vi "SWERVE_DRIVE_ACT.vi"(8 "in Swerve Module States":T4[](array[typedef]) {"Angle"."SIN" format="%13.4f"; "Angle"."COS" format="%13.4f"; "Angle"."VALUE" format="%13.4f"}, 9 "Gyro_Continuous_Rad":dbl, 10 "Swerve Drive Device Reference":T6[](array[typedef]), 11 "in SWERVE_DRIVE_KINEMATICS":T1 {"SavedModuleStates"."Angle"."SIN" format="%13.4f"; "SavedModuleStates"."Angle"."COS" format="%13.4f"; "SavedModuleStates"."Angle"."VALUE" format="%13.4f"; "PrevCoR"."Y" format="%14.3f"; "PrevCoR"."X" format="%14.3f"; "Modules"."Y" format="%14.3f"; "Modules"."X" format="%14.3f"}) -> (3 "out SWERVE_DRIVE_KINEMATICS":T1 {"SavedModuleStates"."Angle"."SIN" format="%13.4f"; "SavedModuleStates"."Angle"."COS" format="%13.4f"; "SavedModuleStates"."Angle"."VALUE" format="%13.4f"; "PrevCoR"."Y" format="%14.3f"; "PrevCoR"."X" format="%14.3f"; "Modules"."Y" format="%14.3f"; "Modules"."X" format="%14.3f"})   [LabVIEW 2019]
uses:
  <vilib>/Rock Robotics/WPI/ThirdParty/JAS_Junk/TrajLib/TypeDef/SWERVE_DRIVE_KINEMATICS.ctl
  <vilib>/Analysis/Matrix/Datatypes/RealMatrix.ctl
  <vilib>/Rock Robotics/WPI/ThirdParty/JAS_Junk/TrajLib/TypeDef/TRANSLATION2D.ctl
  <vilib>/Rock Robotics/WPI/ThirdParty/JAS_Junk/TrajLib/TypeDef/SWERVE_DRIVE_MODULE_STATE.ctl
  <vilib>/Rock Robotics/WPI/ThirdParty/JAS_Junk/TrajLib/TypeDef/ROTATION2D.ctl
  SWERVE_DRIVE_MODULE_TYPDEF.ctl
  <vilib>/Rock Robotics/WPI/MotorControl/WPI_MotorControlDeviceRef.ctl
  <vilib>/Rock Robotics/WPI/MotorControl/WPI_MotorControlType.ctl
  <vilib>/Rock Robotics/SystemInterfaces/DIO/FPGA_DIOPWMChannel.ctl
  <vilib>/Rock Robotics/WPI/PWM/WPI_PWMDeadband.ctl
  <vilib>/Rock Robotics/SystemInterfaces/DIO/FPGA_DIOChannel.ctl
  <vilib>/Rock Robotics/WPI/Encoder/WPI_EncoderDevRef.ctl
  <vilib>/Rock Robotics/SystemInterfaces/Encoder/FPGA_EncoderIdx.ctl
  <vilib>/Rock Robotics/SystemInterfaces/Counter/FPGA_CounterCtrSystemIndex.ctl
  <vilib>/Rock Robotics/WPI/Encoder/WPI_EncoderType.ctl
  Robot Global Data.vi
  Secret_Control_Library_Protected/Secret_Control_Library_Protected.lvlib
  <vilib>/Rock Robotics/WPI/ThirdParty/JAS_Junk/TrajLib/Trajectory_Library.lvlib
  <vilib>/Analysis/Matrix/NI_Matrix.lvlib
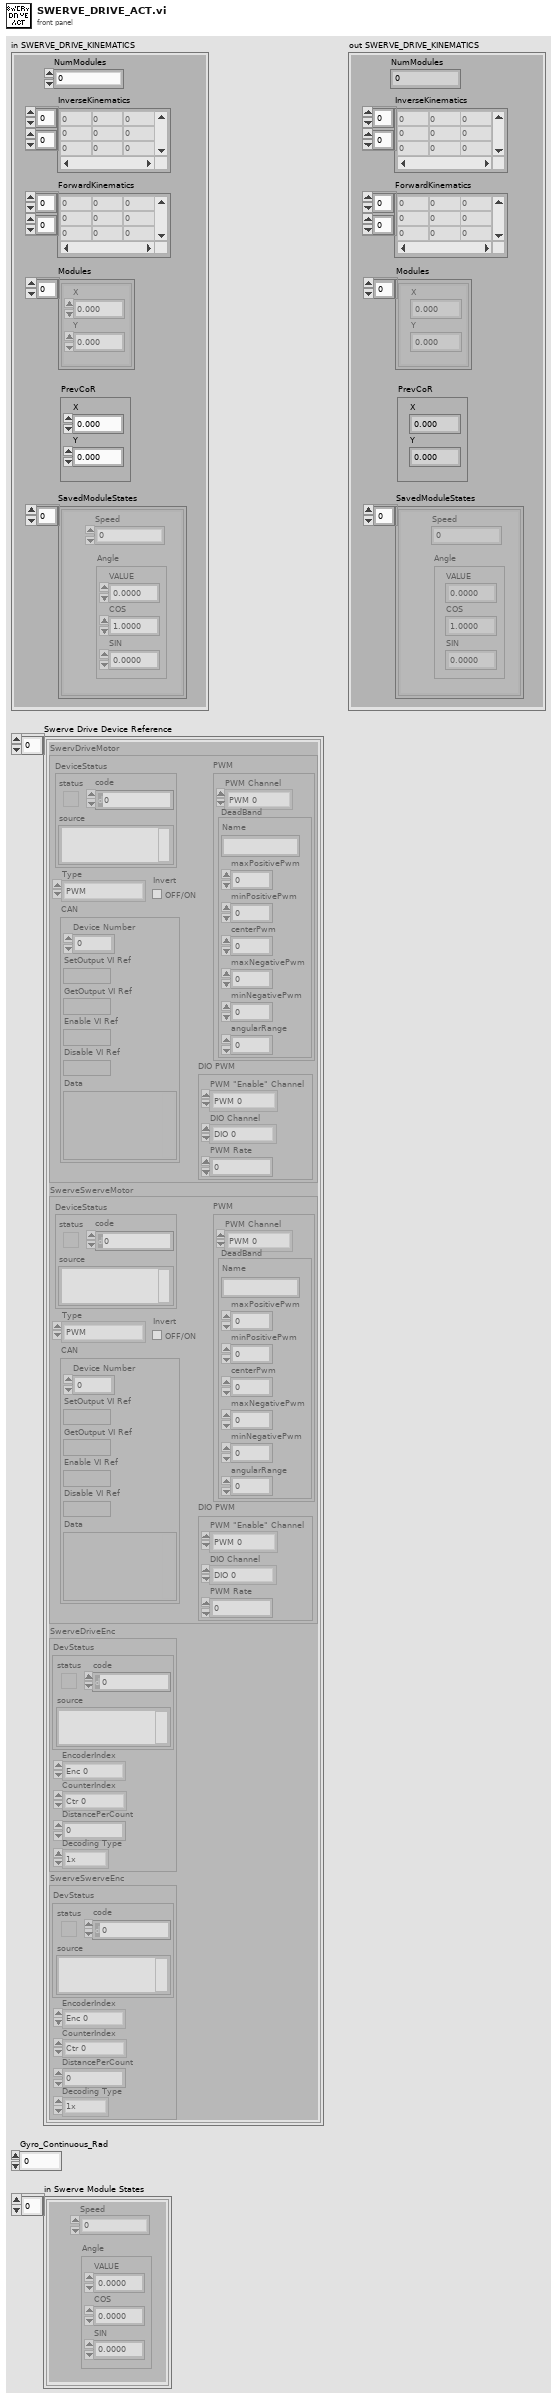
[diagram p1: front panel]
types:
  T1 = typedef "Trajectory_Library.lvlib/SWERVE_DRIVE_KINEMATICS.ctl" = cluster{"NumModules":i32, "InverseKinematics":T2, "ForwardKinematics":T2, "Modules":T3[], "PrevCoR":T3, "SavedModuleStates":T4[]}
  T2 = typedef "NI_Matrix.lvlib/RealMatrix.ctl" = dbl[][]
  T3 = typedef "Trajectory_Library.lvlib/TRANSLATION2D.ctl" = cluster{"X":dbl, "Y":dbl}
  T4 = typedef "Trajectory_Library.lvlib/SWERVE_DRIVE_MODULE_STATE.ctl" = cluster{"Speed":dbl, "Angle":T5}
  T5 = typedef "Trajectory_Library.lvlib/ROTATION2D.ctl" = cluster{"VALUE":dbl, "COS":dbl, "SIN":dbl}
  T6 = typedef "SWERVE_DRIVE_MODULE_TYPDEF.ctl" = cluster{"SwervDriveMotor":T7, "SwerveSwerveMotor":T7, "SwerveDriveEnc":T12, "SwerveSwerveEnc":T12}
  T7 = typedef "WPI_MotorControlDeviceRef.ctl" = cluster{"DeviceStatus":errorcluster, "Type":T8, "PWM":cluster{"PWM Channel":T9, "DeadBand":T10}, "CAN":cluster{"Device Number":u8, "SetOutput VI Ref":variant, "GetOutput VI Ref":variant, "Enable VI Ref":variant, "Disable VI Ref":variant, "Data":variant}, "Invert":bool, "DIO PWM":cluster{"PWM \"Enable\" Channel":T9, "DIOChannel":T11, "PWM Rate":dbl}}
  T8 = typedef "WPI_MotorControlType.ctl" = enum16{"PWM", "CAN", "DIO PWM"}
  T9 = typedef "FPGA_DIOPWMChannel.ctl" = enum8{"PWM 0", "PWM 1", "PWM 2", "PWM 3", "PWM 4", "PWM 5", "PWM 6", "PWM 7", "PWM 8", "PWM 9", "PWM MXP 0", "PWM MXP 1", "PWM MXP 2", "PWM MXP 3", "PWM MXP 4", "PWM MXP 5", "PWM MXP 6", "PWM MXP 7", "PWM MXP 8", "PWM MXP 9", "Invalid"}
  T10 = typedef "WPI_PWMDeadband.ctl" = cluster{"Name":string, "maxPositivePwm":i32, "minPositivePwm":i32, "centerPwm":i32, "maxNegativePwm":i32, "minNegativePwm":i32, "angularRange":u16}
  T11 = typedef "FPGA_DIOChannel.ctl" = enum8{"DIO 0", "DIO 1", "DIO 2", "DIO 3", "DIO 4", "DIO 5", "DIO 6", "DIO 7", "DIO 8", "DIO 9", "DIO MXP 0", "DIO MXP 1", "DIO MXP 2", "DIO MXP 3", "DIO MXP 4", "DIO MXP 5", "DIO MXP 6", "DIO MXP 7", "DIO MXP 8", "DIO MXP 9", "DIO MXP 10", "DIO MXP 11", "DIO MXP 12", "DIO MXP 13", "DIO MXP 14", "DIO MXP 15", "SPI Port CS1", "SPI Port CS2", "SPI Port CS3", "SPI Port MISO", "SPI Port MOSI", "Invalid"}
  T12 = typedef "WPI_EncoderDevRef.ctl" = cluster{"DevStatus":errorcluster, "EncoderIndex":T13, "CounterIndex":T14, "DistancePerCount":dbl, "Decoding Type":T15}
  T13 = typedef "FPGA_EncoderIdx.ctl" = enum8{"Enc 0", "Enc 1", "Enc 2", "Enc 3", "Enc 4", "Enc 5", "Enc 6", "Enc 7", "Invalid"}
  T14 = typedef "FPGA_CounterCtrSystemIndex.ctl" = enum8{"Ctr 0", "Ctr 1", "Ctr 2", "Ctr 3", "Ctr 4", "Ctr 5", "Ctr 6", "Ctr 7", "Invalid"}
  T15 = typedef "WPI_EncoderType.ctl" = enum16{"1x", "2x", "4x"}
  T16 = typedef "Trajectory_Library.lvlib/CHASSIS_SPEEDS.ctl" = cluster{"vX":dbl, "vY":dbl, "vOmega":dbl}
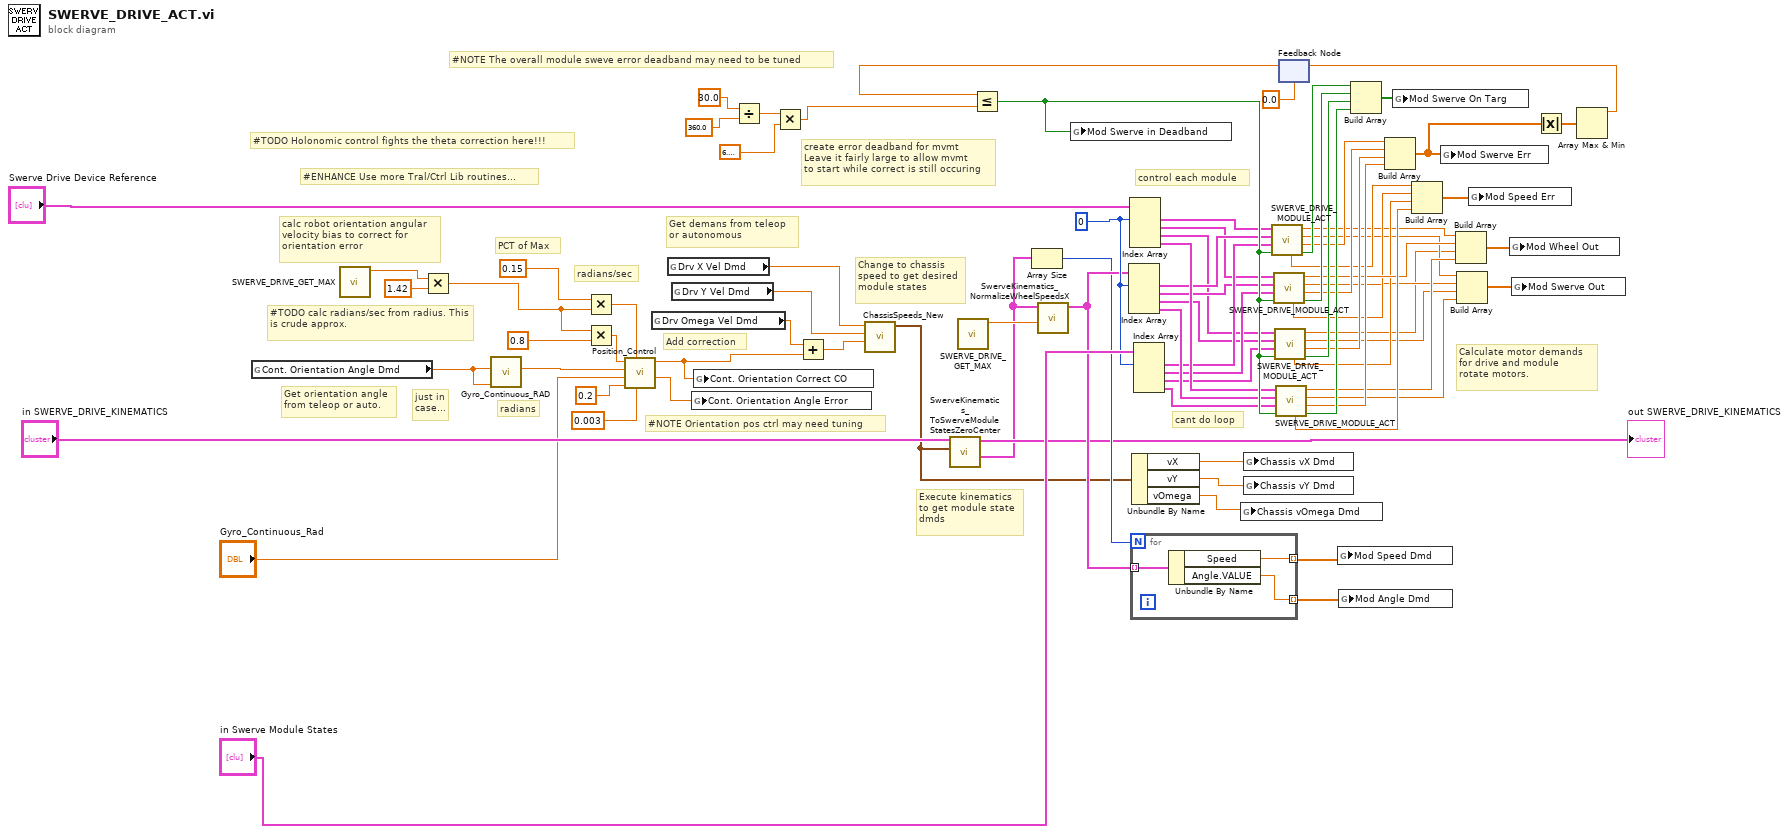
[diagram p0: block diagram]
diagram:
  w36 = 0 ("index")
  # "#NOTE The overall module sweve error deadband may need to be tuned"
  # "create error deadband for mvmt\nLeave it fairly large to allow mvmt\nto start while correct is still occuring"
  # "#TODO Holonomic control fights the theta correction here!!!"
  # "Calculate motor demands\nfor drive and module \nrotate motors."
  # "Execute kinematics\nto get module state\ndmds"
  # "Get orientation angle\nfrom teleop or auto."
  # "Add correction"
  # "Get demans from teleop\nor autonomous"
  # "#ENHANCE Use more Tral/Ctrl Lib routines..."
  # "just in\ncase..."
  # "#TODO calc radians/sec from radius. This is crude approx."
  # "PCT of Max"
  # "#NOTE Orientation pos ctrl may need tuning"
  # "cant do loop"
  # "control each module"
  # "Change to chassis \nspeed to get desired\nmodule states"
  # "radians/sec"
  # "radians"
  # "calc robot orientation angular\nvelocity bias to correct for\norientation error"
  n1 = global read "Robot Global Data.vi" "Cont. Orientation Angle Dmd"() -> (w71:dbl)
  n2 = call "SWERVE_DRIVE_GET_MAX.vi"() -> ("Max Wheel Vel (Meter/Sec)"=w62:dbl)  [unwired: 10 in, 1 out]
  n3 = Multiply(x=w62, y=1.42) -> (x*y=w64:dbl)
  n4 = call "Gyro_Continuous_RAD.vi"("GyroInitial"=w71, "GyroInput"=w71) -> ("GyroContinuous"=w72:dbl)  [unwired: 9 in]
  n5 = Multiply(x=0.15, y=w64) -> (x*y=w1:dbl)
  n6 = Multiply(x=w64, y=0.8) -> (x*y=w43:dbl)
  n7 = call "Position_Control.vi"("ErrDeadband"=0.003, "MinOutput"=w1, "ErrThreshold"=0.2, "CurrentPosition"="Gyro_Continuous_Rad", "TargetPosition"=w72, "MaxOutput"=w43) -> ("PositionError"=w46:dbl, "Output"=w45:dbl)  [unwired: 3 in, 1 out]
  n8 = global read "Robot Global Data.vi" "Drv Omega Vel Dmd"() -> (w5:dbl)
  n9 = global read "Robot Global Data.vi" "Drv X Vel Dmd"() -> (w6:dbl)
  n10 = global read "Robot Global Data.vi" "Drv Y Vel Dmd"() -> (w7:dbl)
  n11 = global write "Robot Global Data.vi" "Cont. Orientation Angle Error"(w46) -> ()
  n12 = global write "Robot Global Data.vi" "Cont. Orientation Correct CO"(w45) -> ()
  n13 = Divide(x=30.0, y=360.0) -> (x/y=w76:dbl)
  n14 = Multiply(x=w76, y=6.283185307179586) -> (x*y=w80:dbl)
  n15 = Add(x=w5, y=w45) -> (x+y=w37:dbl)
  n16 = call <vilib>:"ChassisSpeeds_New.vi"("vAngular"=w37, "vY"=w7, "vX"=w6) -> ("CHASSIS"=w11:T16)  [unwired: 8 in]
  n17 = call <vilib>:"SwerveKinematics_ToSwerveModuleStatesZeroCenter.vi"("ChassisSpeeds"=w11, "in SWERVE_DRIVE_KINEMATICS"="in SWERVE_DRIVE_KINEMATICS") -> ("ModuleStates"=w8:T4[], "out SWERVE_DRIVE_KINEMATICS"=→"out SWERVE_DRIVE_KINEMATICS":T1)  [unwired: 8 in]
  n18 = call "SWERVE_DRIVE_GET_MAX.vi"() -> ("Max Wheel Vel (Meter/Sec)"=w10:dbl)  [unwired: 10 in, 1 out]
  n19 = Array Size(array=w8) -> (size(s)=w15:i32)
  n20 = call <vilib>:"SwerveKinematics_NormalizeWheelSpeedsX.vi"("AttainableMaxSpeed"=w10, "in WheelStates"=w8) -> ("out WheelStates"=w22:T4[])  [unwired: 9 in]
  n21 = Index Array(array=w22, index #1=w36) -> (element #1=w23:T4, element #2=w24:T4, element #3=w25:T4, element #4=w41:T4)  [unwired: 3 in]
  n22 = Index Array(array="Swerve Drive Device Reference", index #1=w36) -> (element #1=w19:T6, element #2=w20:T6, element #3=w21:T6, element #4=w40:T6)  [unwired: 3 in]
  n23 = for {
    N: w15 -> [_]
    tunnel: w22 -> [w83] mode=indexing
    tunnel: [w82] -> w16 mode=indexing
    tunnel: [w81] -> w17 mode=indexing
    n24 = Unbundle By Name(w83) -> ("Speed"=w81:dbl, "Angle.VALUE"=w82:dbl)
  }
  n25 = Unbundle By Name(w11) -> ("vX"=w12:dbl, "vY"=w13:dbl, "vOmega"=w14:dbl)
  n26 = Index Array(array="in Swerve Module States", index #1=w36) -> (element #1=w26:T4, element #2=w27:T4, element #3=w28:T4, element #4=w42:T4)  [unwired: 3 in]
  n27 = global write "Robot Global Data.vi" "Chassis vOmega Dmd"(w14) -> ()
  n28 = global write "Robot Global Data.vi" "Chassis vX Dmd"(w12) -> ()
  n29 = global write "Robot Global Data.vi" "Chassis vY Dmd"(w13) -> ()
  n30 = feedback #1(0.0) -> (w69:dbl)
  n31 = Less Or Equal?(x=w69, y=w80) -> (x <= y?=w70:bool)
  n32 = global write "Robot Global Data.vi" "Mod Swerve in Deadband"(w70) -> ()
  n33 = call "SWERVE_DRIVE_MODULE_ACT.vi"("SwervePosInDeadband"=w70, "Swerve Sense"=w26, "Swerve Dmd"=w23, "Swerve Module TypDef"=w19) -> ("SwerveOnTarget"=w58:bool, "SwervePosError"=w52:dbl, "Swerve Motor Dmd"=w32:dbl, "Wheel Motor Dmd"=w29:dbl, "WheelSpeedErr"=w48:dbl)  [unwired: 3 in]
  n34 = call "SWERVE_DRIVE_MODULE_ACT.vi"("SwervePosInDeadband"=w70, "Swerve Sense"=w27, "Swerve Dmd"=w24, "Swerve Module TypDef"=w20) -> ("SwerveOnTarget"=w59:bool, "SwervePosError"=w53:dbl, "Swerve Motor Dmd"=w33:dbl, "Wheel Motor Dmd"=w51:dbl, "WheelSpeedErr"=w49:dbl)  [unwired: 3 in]
  n35 = call "SWERVE_DRIVE_MODULE_ACT.vi"("SwervePosInDeadband"=w70, "Swerve Sense"=w28, "Swerve Dmd"=w25, "Swerve Module TypDef"=w21) -> ("SwerveOnTarget"=w60:bool, "SwervePosError"=w54:dbl, "Swerve Motor Dmd"=w34:dbl, "Wheel Motor Dmd"=w30:dbl, "WheelSpeedErr"=w50:dbl)  [unwired: 3 in]
  n36 = call "SWERVE_DRIVE_MODULE_ACT.vi"("SwervePosInDeadband"=w70, "Swerve Sense"=w42, "Swerve Dmd"=w41, "Swerve Module TypDef"=w40) -> ("SwerveOnTarget"=w61:bool, "SwervePosError"=w55:dbl, "Swerve Motor Dmd"=w39:dbl, "Wheel Motor Dmd"=w38:dbl, "WheelSpeedErr"=w56:dbl)  [unwired: 3 in]
  n37 = global write "Robot Global Data.vi" "Mod Speed Dmd"(w17) -> ()
  n38 = global write "Robot Global Data.vi" "Mod Angle Dmd"(w16) -> ()
  n39 = Build Array(w58, w59, w60, w61) -> (w57:bool[])
  n40 = Build Array(w52, w53, w54, w55) -> (w66:dbl[])
  n41 = global write "Robot Global Data.vi" "Mod Swerve On Targ"(w57) -> ()
  n42 = Build Array(w48, w49, w50, w56) -> (w47:dbl[])
  n43 = global write "Robot Global Data.vi" "Mod Swerve Err"(w66) -> ()
  n44 = Build Array(w29, w51, w30, w38) -> (w31:dbl[])
  n45 = Build Array(w32, w33, w34, w39) -> (w35:dbl[])
  n46 = global write "Robot Global Data.vi" "Mod Speed Err"(w47) -> ()
  n47 = global write "Robot Global Data.vi" "Mod Wheel Out"(w31) -> ()
  n48 = global write "Robot Global Data.vi" "Mod Swerve Out"(w35) -> ()
  n49 = Absolute Value(x=w66) -> (abs(x)=w65:dbl[])
  n50 = Array Max & Min(array=w65) -> (max value=w67:dbl)  [unwired: 3 out]
  n51 = feedback-in #1(w67) -> ()
